vi "KickToPassReceiverTactic.vi"(7 "first call":bool, 8 "error in (no error)":errorcluster, 9 "Robot":refnum<class "Robot.lvclass">, 10 "Game in":refnum<class "Game.lvclass">, 11 "KickToPassReceiverTactic in":refnum<class "KickToPassReceiverTactic.lvclass">) -> (0 "error out":errorcluster, 2 "Robot out":refnum<class "Robot.lvclass">, 3 "KickToPassReceiverTactic out":refnum<class "KickToPassReceiverTactic.lvclass">)   [LabVIEW 2023, in "KickToPassReceiverTactic.lvclass"]
uses:
  KickToPassReceiverTactic.lvclass
  C:/Users/roboi/Downloads/VSS_AI-Larc2023 - Copia (2)/Tactic_class/Tactic.lvclass
  Robot_class/Robot.lvclass
  C:/Users/roboi/Downloads/VSS_AI-Larc2023 - Copia (2)/Object_class/Object.lvclass
  Game_class/Game.lvclass
  Robot_class/Robot.lvclass/Robot.ctl
  Robot_class/tactics.ctl
  Team_class/OffensivePlay.ctl
  Tactic_class/Tactic.lvclass/Tactic.ctl
  Game_class/Game.lvclass/Game.ctl
  Parameters_class/Parameters.lvclass/Parameters.ctl
  Team_class/Team.lvclass/Team.ctl
  Robot_class/roles.ctl
  Object_class/Object.lvclass/Object.ctl
  Skillbook_class/Skillbook.lvclass/Skillbook.ctl
  Events_class/Events.lvclass/Events.ctl
  Robot_class/Read role.vi
  Object_class/Read x.vi
  Object_class/Read y.vi
  Events_class/Read kick.vi
  Events_class/Read touch.vi
  Game_class/Read EventsRef.vi
  Game_class/Read OffensiveTeam.vi
  Team_class/Read OffensivePlay.vi
  Skillbook_class/Read KickToSkill.vi
  Skillbook_class/Read HaltSkill.vi
  Game_class/Read Parameters.lvclass.vi
  Game_class/Read Utilities.lvclass.vi
  Game_class/Read BallRef.vi
  Game_class/Read FieldRef.vi
  Team_class/Read RobotRef.vi
  Parameters_class/Read AttakingOurselves.vi
  Tactic_class/Read Skillbook.vi
  Robot_class/Write tactic.vi
  Ally_class/Ally.lvclass
  C:/Users/roboi/Downloads/VSS_AI-Larc2023 - Copia (2)/Team_class/Team.lvclass
  Ball_class/Ball.lvclass
  Parameters_class/Parameters.lvclass
  Utilities_class/Utilities.lvclass
  Field_class/Field.lvclass
  Skillbook_class/Skillbook.lvclass
  Events_class/Events.lvclass
  KickToSkill_class/KickToSkill.lvclass
  HaltSkill_class/HaltSkill.lvclass
panel:
  out "x .or. y?":bool
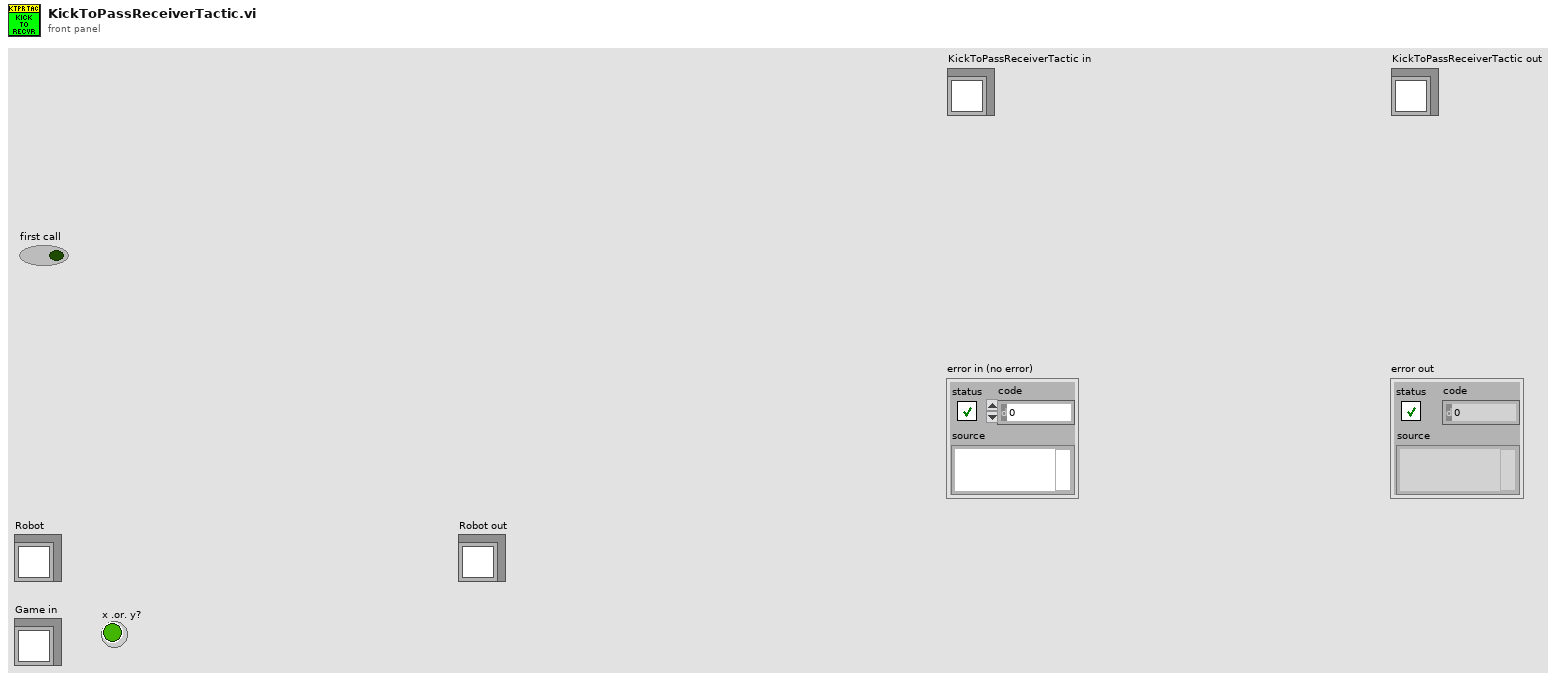
[diagram p1: front panel]
types:
  T1 = typedef "OffensivePlay.ctl" = enum16{"TableWithStriker", "TableWith2ndStrikerPlay", "PrepareDoublePass", "PrepareRollToPass", "SimplePass", "PreparePass", "PassToStriker", "BallOutOfField", "PassTo2ndStriker", "StopOffensive", "Prepare Penalty Enemy", "EnemyPossessionAtEnemyField", "EnemyPossesionAtOurField", "TestPlay", "PreparePenaltyAlly", "KickPenaltyAlly", "PrepareKickoffAlly", "PrepareKickoffEnemy", "IndirectEnemy", "DirectEnemy", "NormalGame", "DirectKick", "Pass", "Halt", "Timeout", "PassPlay", "PenaltyEnemy"}
  T2 = typedef "tactics.ctl" = enum16{"ReceivePassInFuturePoint", "Roller", "PrepareRollToPassRollerGoTo", "PrepareRollToPassReceiverGoTo", "WaitRoll", "PositionToRoll", "PenaltyAttacker", "PassObserver", "PenaltyDefense", "TableReceiverTactic", "Test", "DefendGoal", "Marker", "FollowAttacker", "DefendArea", "Shoot", "AttackerAimGoal", "AttackerBallOutOfField", "AttackerBlock", "AttackerStop", "Duelist", "Halt", "ZigZag", "GoTo", "Timeout", "KickToPassReceiver", "PositionToReceivePass", "DefendAreaVSS", "DefendGoalVSS", "KickVSS", "AttackVSS", "DispBallVSS", "PenaltyAttackVSS", "WaitPass"}
  T3 = typedef "roles.ctl" = enum16{"BallChallengerAttackerVSS", "NormalAttackerVSS", "AttackerAimGoalVSS", "DefenderAreaVSS", "KeeperVSS", "Tabler", "TableFinalizer", "PrepareRollToPassRoller", "PrepareRollToPassReceiver", "SimplePassRoll", "SimplePassRollReceiver", "PenaltyDefense", "PreparePassReceiver 2", "PreparePassReceiver 1", "PassObserver", "Timeout", "Goto", "ZigZag", "None", "BallOutOfField", "DefenderArea", "Duelist", "AttackerStop", "FollowAttacker", "KeeperRole", "KickPenalty", "AttackerAimGoal", "AttackerBlock", "Marker", "Halt", "Shoot", "PassKicker", "PassReceiver", "TestRole", "PenaltyAttacker"}
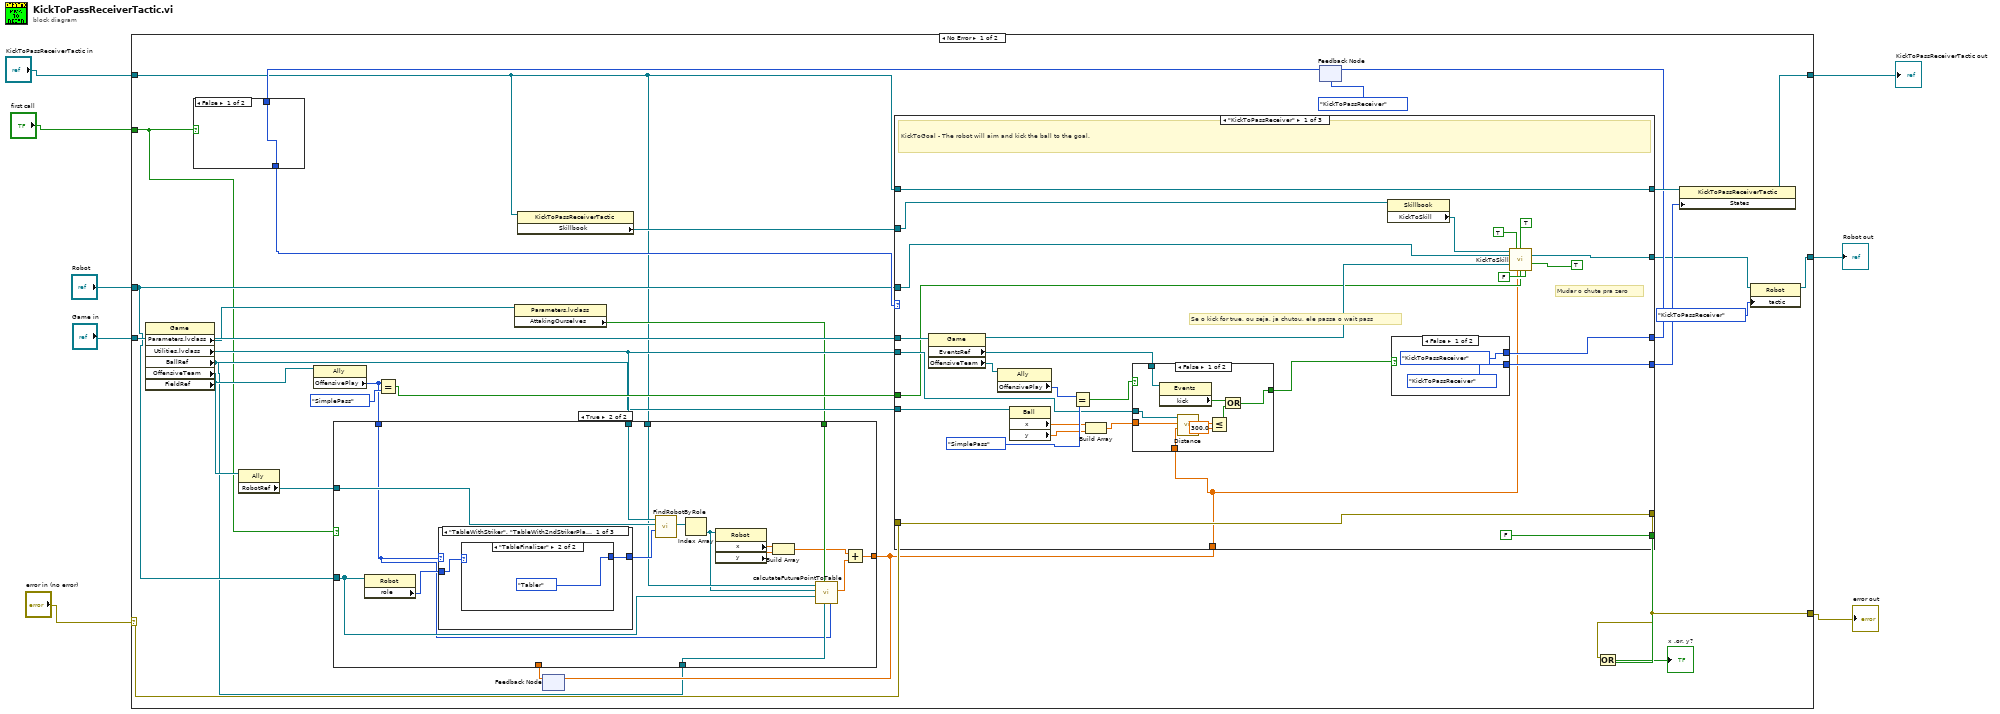
[diagram p0: block diagram]
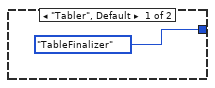
[diagram p3: hidden frame]
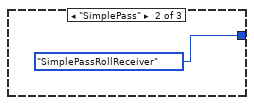
[diagram p4: hidden frame]
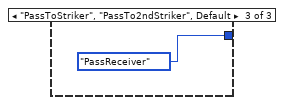
[diagram p5: hidden frame]
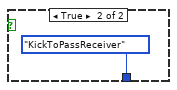
[diagram p6: hidden frame]
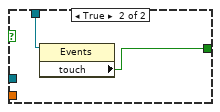
[diagram p7: hidden frame]
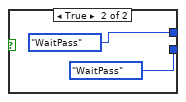
[diagram p8: hidden frame]
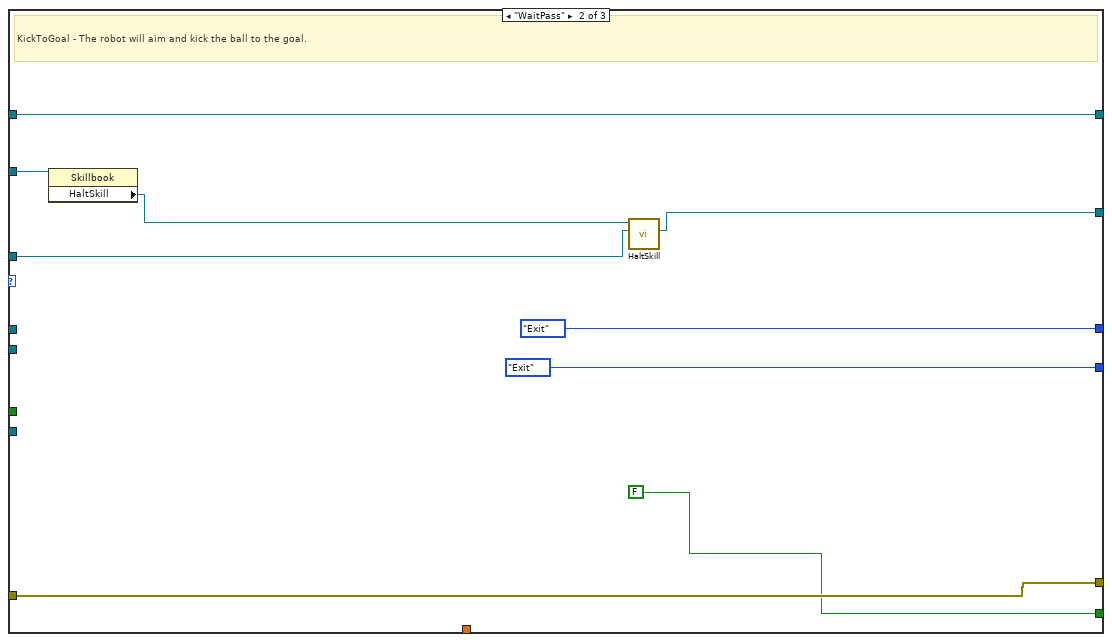
[diagram p9: hidden frame]
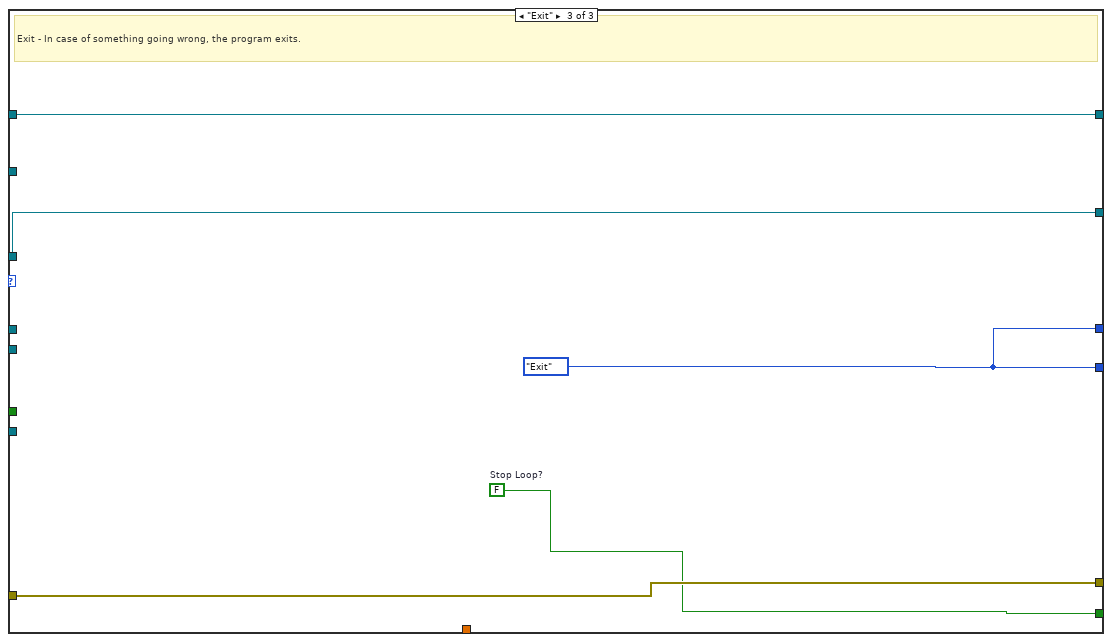
[diagram p10: hidden frame]
diagram:
  n1 = case shown="No Error" "error in (no error)" {
    selector: "error in (no error)" -> [w32 w123]
    tunnel: [w33 w123] -> w2
    tunnel: [w34 w122] -> w3
    tunnel: "KickToPassReceiverTactic in" -> [w10 w122]
    tunnel: "Robot" -> [w15 w121]
    tunnel: "Game in" -> [w31 _]
    tunnel: [w23 w121] -> w6
    tunnel: "first call" -> [w9 _]
    frame No Error {
      n2 = property class="Game" props=["Parameters.lvclass", "Utilities.lvclass", "BallRef", "OffensiveTeam", "FieldRef"](reference=w31) -> ("Parameters.lvclass"=w12:refnum<class "Parameters.lvclass">, "Utilities.lvclass"=w17:refnum<class "Utilities.lvclass">, "BallRef"=w13:refnum<class "Ball.lvclass">, "OffensiveTeam"=w20:refnum<class "Ally.lvclass">)  [unwired: 1 in, 3 out]
      n3 = property class="Ally"(reference=w20) -> ("RobotRef"=w30:refnum<class "Robot.lvclass">[])  [unwired: 1 in, 2 out]
      n4 = property class="Ally"(reference=w20) -> ("OffensivePlay"=w16:T1)  [unwired: 1 in, 2 out]
      n5 = Equal?(x=w16, y=OffensivePlay."SimplePass" ("OffensivePlay")) -> (x = y?=w19:bool)
      n6 = property class="Parameters.lvclass"(reference=w12) -> ("AttakingOurselves"=w11:bool)  [unwired: 1 in, 2 out]
      n7 = property class="KickToPassReceiverTactic"(reference=w10) -> ("Skillbook"=w36:refnum<class "Skillbook.lvclass">)  [unwired: 1 in, 2 out]
      n8 = feedback #1() -> (w18:dbl[])  [unwired: 1 in]
      n9 = case shown="True" w9 {
        tunnel: w30 -> [_ w55]
        tunnel: w18 -> [w39 _]
        tunnel: w17 -> [_ w54]
        tunnel: w16 -> [_ w40]
        tunnel: w15 -> [_ w42]
        tunnel: [w39 w50] -> w14
        tunnel: w13 -> [_ w41]
        tunnel: w11 -> [_ w46]
        tunnel: w10 -> [_ w45]
        frame False {
        }
        frame True {
          n10 = property class="Robot"(reference=w42) -> ("role"=w48:T3)  [unwired: 1 in, 2 out]
          n11 = case shown="\"TableWithStriker\", \"TableWith2ndStrikerPlay\"" w40 {
            tunnel: [w57 roles."SimplePassRollReceiver" ("role") roles."PassReceiver" ("role")] -> w49
            tunnel: w48 -> [w56 _ _]
            frame "TableWithStriker", "TableWith2ndStrikerPlay" {
              n12 = case shown="\"TableFinalizer\"" w56 {
                tunnel: [roles."TableFinalizer" ("role") roles."Tabler" ("role")] -> w57
                frame "Tabler", Default {
                }
                frame "TableFinalizer" {
                }
              }
            }
            frame "SimplePass" {
            }
            frame "PassToStriker", "PassTo2ndStriker", Default {
            }
          }
          n13 = call "FindRobotByRole.vi"("role"=w49, "RobotRef"=w55, "Utilities in"=w54) -> ("Robots"=w53:refnum<class "Robot.lvclass">[])  [unwired: 6 in, 2 out]
          n14 = Index Array(array=w53) -> (element=w43:refnum<class "Robot.lvclass">)  [unwired: 1 in]
          n15 = property class="Robot"(reference=w43) -> ("x"=w52:dbl, "y"=w51:dbl)  [unwired: 1 in, 2 out]
          n16 = Build Array(w52, w51) -> (w44:dbl[])
          n17 = call "calcutateFuturePointToTable.vi"("OffensivePlay"=w40, "BallRef"=w41, "AttackingOurselves?"=w46, "Robot that\nmake the pass"=w42, "Robot that will\nreceive the pass"=w43, "KickToPassReceiverTactic in"=w45) -> ("Array to Receiver trajectory"=w47:dbl[])  [unwired: 3 in, 2 out]
          n18 = Add(x=w44, y=w47) -> (x+y=w50:dbl[])
        }
      }
      n19 = feedback-in #1(w14) -> ()
      n20 = feedback #2(enum16{"KickToPassReceiver", "WaitPass", "Exit"}."KickToPassReceiver" ("States")) -> (w26:enum16{"KickToPassReceiver", "WaitPass", "Exit"})
      n21 = case shown="False" w9 {
        tunnel: [w62 enum16{"KickToPassReceiver", "WaitPass", "Exit"}."KickToPassReceiver" ("States")] -> w27
        tunnel: w26 -> [w62 _]
        frame False {
        }
        frame True {
        }
      }
      n22 = case shown="\"KickToPassReceiver\"" w27 {
        tunnel: [FALSE ("Stop Loop?") FALSE ("Stop Loop?") w117] -> w38
        tunnel: w32 -> [w90 w109 w120]
        tunnel: [w90 w109 w120] -> w33
        tunnel: w36 -> [w89 w114 _]
        tunnel: w15 -> [w84 w115 w118]
        tunnel: [w87 w112 w118] -> w24
        tunnel: [w88 w111 w119] -> w35
        tunnel: w10 -> [w88 w111 w119]
        tunnel: w31 -> [w83 _ _]
        tunnel: [w81 enum16{"KickToPassReceiver", "WaitPass", "Exit"}."Exit" ("States") w116] -> w29
        tunnel: [w80 enum16{"KickToPassReceiver", "WaitPass", "Exit"}."Exit" ("States") w116] -> w28
        tunnel: w13 -> [w70 _ _]
        tunnel: w17 -> [w66 _ _]
        tunnel: w19 -> [w65 _ _]
        tunnel: w14 -> [w64 _ _]
        frame "KickToPassReceiver" {
          # "Se o kick for true, ou seja, ja chutou, ele passa o wait pass"
          # "Mudar o chute pra zero"
          # "KickToGoal - The robot will aim and kick the ball to the goal."
          n23 = property class="Game"(reference=w83) -> (reference out=w82:refnum<class "Game.lvclass">, "EventsRef"=w74:refnum<class "Events.lvclass">, "OffensiveTeam"=w72:refnum<class "Ally.lvclass">)  [unwired: 1 in, 1 out]
          n24 = property class="Ally"(reference=w72) -> ("OffensivePlay"=w77:T1)  [unwired: 1 in, 2 out]
          n25 = property class="Ball"(reference=w70) -> ("x"=w69:dbl, "y"=w68:dbl)  [unwired: 1 in, 2 out]
          n26 = Equal?(x=w77, y=OffensivePlay."SimplePass" ("OffensivePlay")) -> (x = y?=w75:bool)
          n27 = Build Array(w69, w68) -> (w67:dbl[])
          n28 = case shown="False" w75 {
            tunnel: w74 -> [w100 w102]
            tunnel: [w98 w101] -> w73
            tunnel: w64 -> [w97 _]
            tunnel: w67 -> [w96 _]
            tunnel: w66 -> [w92 _]
            frame False {
              n29 = property class="Events"(reference=w100) -> ("kick"=w99:bool)  [unwired: 1 in, 2 out]
              n30 = call "Distance.vi"("P1"=w97, "P2"=w96, "Utilities in"=w92) -> ("Distance"=w95:dbl)  [unwired: 6 in, 2 out]
              n31 = Less Or Equal?(x=w95, y=300.0) -> (x <= y?=w93:bool)
              n32 = Or(x=w99, y=w93) -> (x .or. y?=w98:bool)
            }
            frame True {
              n33 = property class="Events"(reference=w102) -> ("touch"=w101:bool)  [unwired: 1 in, 2 out]
            }
          }
          n34 = property class="Skillbook"(reference=w89) -> ("KickToSkill"=w85:refnum<class "KickToSkill.lvclass">)  [unwired: 1 in, 2 out]
          n35 = case shown="False" w73 {
            tunnel: [enum16{"KickToPassReceiver", "WaitPass", "Exit"}."KickToPassReceiver" ("States") enum16{"KickToPassReceiver", "WaitPass", "Exit"}."WaitPass" ("States")] -> w81
            tunnel: [enum16{"KickToPassReceiver", "WaitPass", "Exit"}."KickToPassReceiver" ("States") enum16{"KickToPassReceiver", "WaitPass", "Exit"}."WaitPass" ("States")] -> w80
            frame False {
            }
            frame True {
            }
          }
          n36 = call "KickToSkill.vi"("KickToSkill in"=w85, "use criteria?"=TRUE, "chipKick ?"=TRUE, "Robot"=w84, "Game"=w82, "calculate force?"=TRUE, "Target"=w64, "KickForce 0?"=w65, "Pass?"=FALSE) -> ("Robot out"=w87:refnum<class "Robot.lvclass">)  [unwired: 4 in, 2 out]
        }
        frame "WaitPass" {
          # "KickToGoal - The robot will aim and kick the ball to the goal."
          n37 = property class="Skillbook"(reference=w114) -> ("HaltSkill"=w113:refnum<class "HaltSkill.lvclass">)  [unwired: 1 in, 2 out]
          n38 = call-dynamic "HaltSkill.vi"("Robot"=w115, "HaltSkill in"=w113) -> ("Robot out"=w112:refnum<class "Robot.lvclass">)  [unwired: 7 in, 2 out]
        }
        frame "Exit" {
          w116 = enum16{"KickToPassReceiver", "WaitPass", "Exit"}."Exit" ("States")
          w117 = FALSE  # Stop Loop?
          # "Exit - In case of something going wrong, the program exits."
        }
      }
      n39 = feedback-in #2(w28) -> ()
      n40 = Or(x=w33, y=w38) -> (x .or. y?=→"x .or. y?":bool)
      n41 = property class="KickToPassReceiverTactic"(reference=w35, "States"=w29) -> (reference out=w34:refnum<class "KickToPassReceiverTactic.lvclass">)  [unwired: 1 in, 1 out]
      n42 = property class="Robot"(reference=w24, "tactic"=tactics."KickToPassReceiver") -> (reference out=w23:refnum<class "Robot.lvclass">)  [unwired: 1 in, 1 out]
    }
    frame Error {
    }
  }
  "error out" <- w2
  "KickToPassReceiverTactic out" <- w3
  "Robot out" <- w6
